vi "SelectPath.vi"() -> ()   [LabVIEW 2018, in "PNA-X.lvlib"]
uses:
  PNA-X.lvlib
panel:
  in  "Tab Control":enum32{"RF PATH", "IF PATH"}(tab)
  out "String":string
  out "VISA Out":refnum<visa-resource-name>="GPIB1::16::INSTR"
  out "error out":errorcluster
  in  "stop":bool
  in  "OK Button":bool
  in  "error in":errorcluster
  in  "Box 1":string(combo)="Path Configuration" caption="Please Select Combiner's Value"
  in  "VNA Visa":refnum<visa-resource-name>="GPIB1::16::INSTR"
  # "Please Select VNA Address"
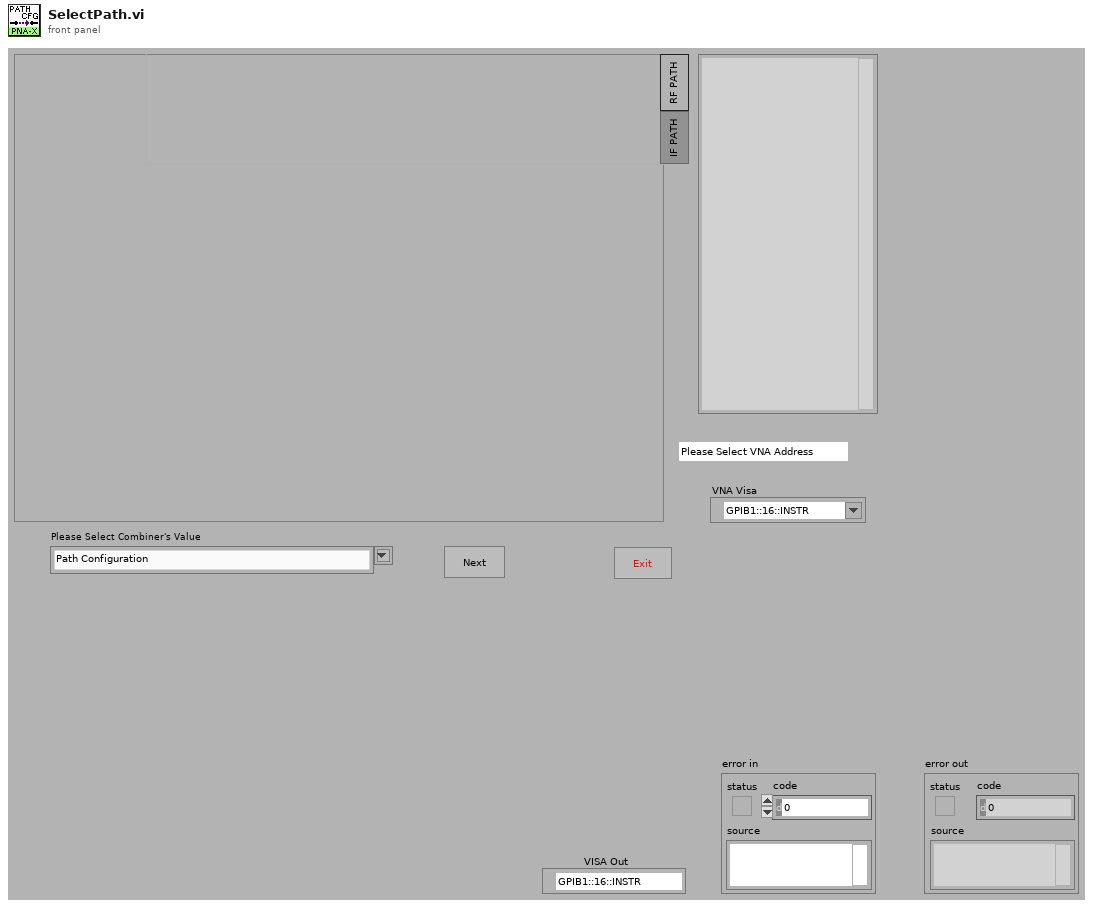
[diagram p1: front panel]
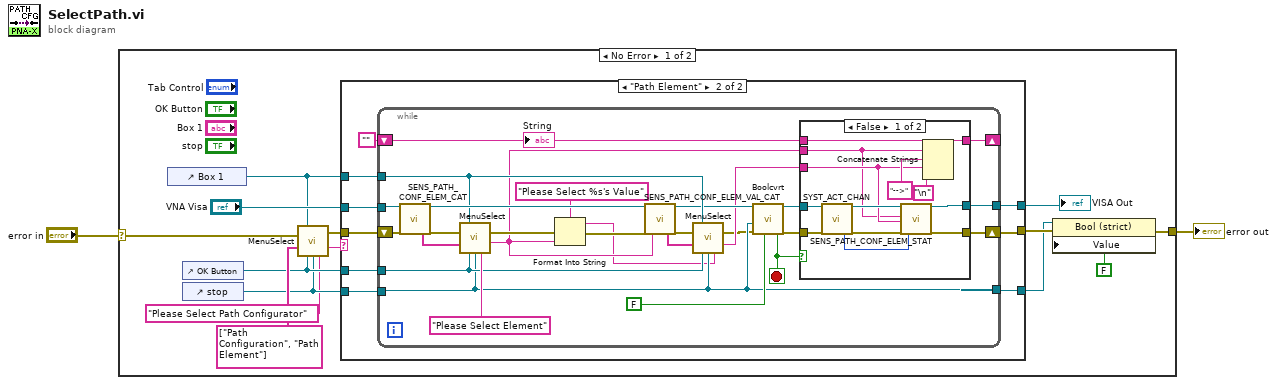
[diagram p0: block diagram]
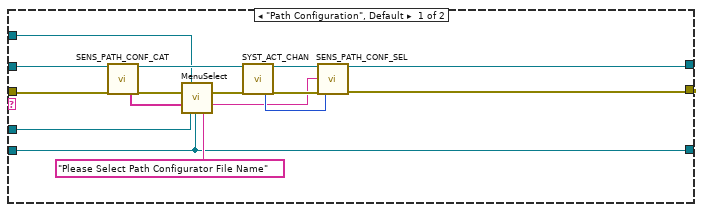
[diagram p2: hidden frame]
diagram:
  n1 = case shown="No Error" "error in" {
    selector: "error in" -> [w4 w84]
    tunnel: [w7 w84] -> w2
    frame No Error {
      n2 = control-ref of="Box 1"() -> (w14:refnum<vi>)
      n3 = control-ref of="OK Button"() -> (w12:refnum<vi>)
      n4 = control-ref of="stop"() -> (w11:refnum<vi>)
      n5 = call "MenuSelect.vi"("Combo Bpx"=w14, "error in"=w4, "Data"=string[] ["Path Configuration", "Path Element"], "OK"=w12, "stop"=w11, "Caption"="Please Select Path Configurator") -> ("error out"=w15:errorcluster, "Value"=w9:string)  [unwired: 8 in]
      n6 = case shown="\"Path Element\"" w9 {
        tunnel: "VNA Visa" -> [w32 w41]
        tunnel: [w27 w33] -> w8
        tunnel: [w18 w40] -> w3
        tunnel: w15 -> [w26 w38]
        tunnel: w14 -> [w20 w37]
        tunnel: w12 -> [w22 w36]
        tunnel: w11 -> [w17 w35]
        tunnel: [w17 w34] -> w6
        frame "Path Configuration", Default {
          n7 = call "SENS_PATH_CONF_CAT.vi"("VISA IN"=w32, "error in"=w26) -> ("Data"=w24:string[], "VISA Out"=w31:refnum<visa-resource-name>, "error out"=w25:errorcluster)  [unwired: 14 in, 1 out]
          n8 = call "MenuSelect.vi"("Combo Bpx"=w20, "error in"=w25, "Data"=w24, "OK"=w22, "stop"=w17, "Caption"="Please Select Path Configurator File Name") -> ("error out"=w21:errorcluster, "Value"=w19:string)  [unwired: 8 in]
          n9 = call "SYST_ACT_CHAN.vi"("VISA IN"=w31, "error in"=w21) -> ("Channel"=w28:i32, "VISA Out"=w30:refnum<visa-resource-name>, "error out"=w29:errorcluster)  [unwired: 15 in]
          n10 = call "SENS_PATH_CONF_SEL.vi"("VISA IN"=w30, "FileName"=w19, "error in"=w29, "Channel"=w28) -> ("VISA Out"=w18:refnum<visa-resource-name>, "error out"=w27:errorcluster)  [unwired: 14 in]
        }
        frame "Path Element" {
          n11 = while {
            tunnel: w41 -> [w66]
            tunnel: [w64] -> w40
            shift-right: [w63] -> _
            shift-left: "" -> [w62]
            tunnel: w37 -> [w54]
            tunnel: w36 -> [w53]
            tunnel: w35 -> [w49]
            shift-right: [w65] -> w33
            shift-left: w38 -> [w55]
            tunnel: [w49] -> w34
            stop <- w52 stop-if-true
            n12 = call "SENS_PATH_CONF_ELEM_CAT.vi"("VISA IN"=w66, "error in"=w55) -> ("Data"=w60:string[], "VISA Out"=w58:refnum<visa-resource-name>, "error out"=w61:errorcluster)  [unwired: 14 in, 1 out]
            n13 = call "MenuSelect.vi"("Combo Bpx"=w54, "error in"=w61, "Data"=w60, "OK"=w53, "stop"=w49, "Caption"="Please Select Element") -> ("error out"=w46:errorcluster, "Value"=w44:string)  [unwired: 8 in]
            n14 = Format Into String(format string="Please Select %s's Value", error in=w46, w44) -> (resulting string=w42:string, error out=w45:errorcluster)  [unwired: 1 in]
            n15 = call "SENS_PATH_CONF_ELEM_VAL_CAT.vi"("VISA IN"=w58, "error in"=w45, "Switch"=w44) -> ("Data"=w56:string[], "VISA Out"=w51:refnum<visa-resource-name>, "error out"=w57:errorcluster)  [unwired: 14 in]
            n16 = call "MenuSelect.vi"("Combo Bpx"=w54, "error in"=w57, "Data"=w56, "OK"=w53, "stop"=w49, "Caption"=w42) -> ("error out"=w48:errorcluster, "Value"=w50:string)  [unwired: 8 in]
            n17 = call "Boolcvrt.vi"("ORide"=FALSE, "error in"=w48, "Bool Refnum"=w49) -> ("error out"=w47:errorcluster, "T/F"=w52:bool)  [unwired: 7 in]
            n18 = case shown="False" w52 {
              tunnel: [w80 w81] -> w65
              tunnel: [w79 w82] -> w64
              tunnel: [w78 w83] -> w63
              tunnel: w62 -> [w77 w83]
              tunnel: w47 -> [w71 w81]
              tunnel: w51 -> [w70 w82]
              tunnel: w44 -> [w68 _]
              tunnel: w50 -> [w69 _]
              frame False {
                n19 = call "SYST_ACT_CHAN.vi"("VISA IN"=w70, "error in"=w71) -> ("Channel"=w74:i32, "VISA Out"=w75:refnum<visa-resource-name>, "error out"=w76:errorcluster)  [unwired: 15 in]
                n20 = call "SENS_PATH_CONF_ELEM_STAT.vi"("VISA IN"=w75, "Element"=w68, "Value"=w69, "error in"=w76, "Channel"=w74) -> ("VISA Out"=w79:refnum<visa-resource-name>, "error out"=w80:errorcluster)  [unwired: 13 in]
                n21 = Concatenate Strings(w77, w68, "-->" ("string"), w69, "\n") -> (w78:string)
              }
              frame True {
              }
            }
            "String" <- w62
          }
        }
      }
      "VISA Out" <- w3
      n22 = property class="Bool (strict)"(reference=w6, error in=w8, "Value"=FALSE) -> (error out=w7:errorcluster)  [unwired: 1 out]
    }
    frame Error {
    }
  }
  "error out" <- w2
